vi "WFS Calc Spots Centr Dia Intens.vi"(8 "error in (no error)":errorcluster {"code" format="%.0x"}, 9 "Calculate Diameters (Off)":bool, 10 "Dynamic Noise Cut (On)":bool=TRUE, 11 "instrument handle":refnum<visa-resource-name>) -> (0 "error out":errorcluster {"code" format="%.0x"}, 3 "instrument handle out":refnum<visa-resource-name>)   [LabVIEW 2020]
doc: "This VI calculates the centroids, diameters (optional) and intensities of all spots generated by the lenslets.\n\nData arrays are returned by separate VIs:\nGetSpotCentroids\nGetSpotDiameters\nGetSpotIntensities\n\nNote: This VI is not available in Highspeed Mode!"
uses:
  WFS_32.dll
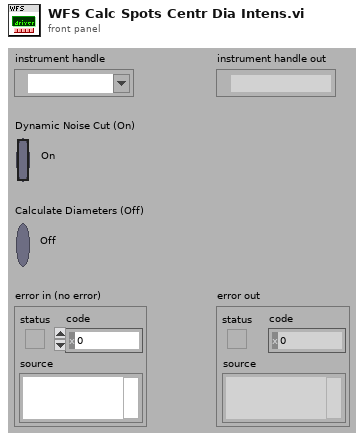
[diagram p1: front panel]
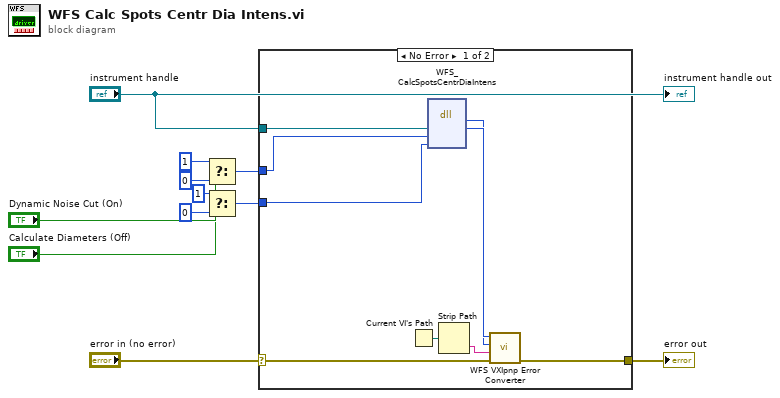
[diagram p0: block diagram]
diagram:
  n1 = Select(t=1, s="Dynamic Noise Cut (On)", f=0) -> (s? t:f=w5:i32)
  n2 = Select(t=1, s="Calculate Diameters (Off)", f=0) -> (s? t:f=w1:i32)
  n3 = case shown="No Error" "error in (no error)" {
    selector: "error in (no error)" -> [w15 w21]
    tunnel: [w14 w21] -> w11
    tunnel: "instrument handle" -> [w19 _]
    tunnel: w5 -> [w13 _]
    tunnel: w1 -> [w12 _]
    frame No Error {
      n4 = Current VI's Path() -> (path=w20:path)
      n5 = dll-call lib="WFS_*.*" fn="WFS_CalcSpotsCentrDiaIntens"("Instrument Handle"=w19, "Dynamic Noise Cut"=w13, "Calculate Diameters"=w12) -> (w17:i32, "Instrument Handle"=w18:u32)  [unwired: 5 in, 2 out]
      n6 = Strip Path(path=w20) -> (name=w16:string)  [unwired: 1 out]
      n7 = call "WFS VXIpnp Error Converter.vi"("error in (no error)"=w15, "Name Of VI (\"\")"=w16, "CVI Error Code (0)"=w17, "instrument handle"=w18) -> ("error out"=w14:errorcluster)  [unwired: 6 in, 1 out]
    }
    frame Error {
    }
  }
  "error out" <- w11
  "instrument handle out" <- "instrument handle"
